vi "valves_pumpsteps.vi"(0 "COM4 in":refnum<k24>, 2 "Pump frequency":dbl=1.0, 3 "Commands in":T1, 5 "error in":errorcluster) -> (6 "COM4 out":refnum<k24>, 8 "error out":errorcluster)   [LabVIEW 2018]
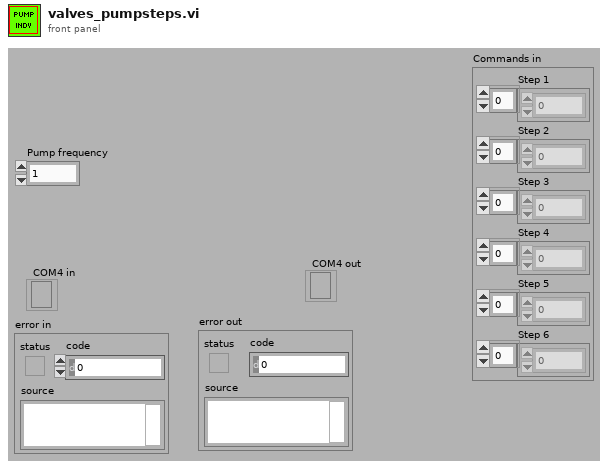
[diagram p1: front panel]
types:
  T1 = cluster{"Step 1":u8[], "Step 2":u8[], "Step 3":u8[], "Step 4":u8[], "Step 5":u8[], "Step 6":u8[]}
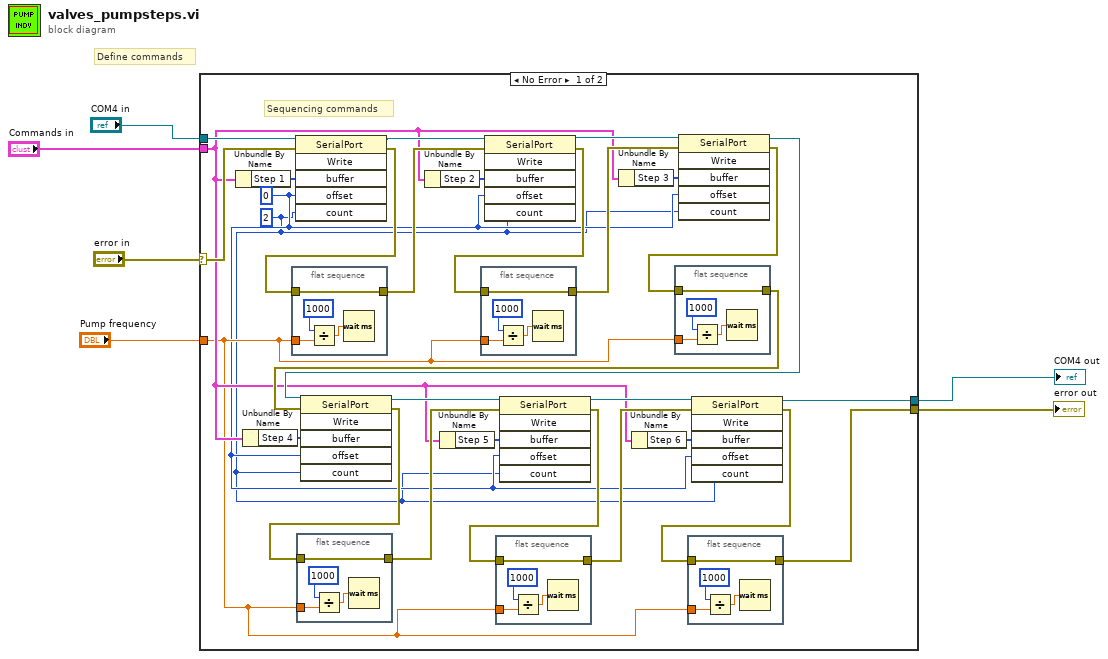
[diagram p0: block diagram]
diagram:
  # "Define commands"
  n1 = case shown="No Error" "error in" {
    selector: "error in" -> [w35 w62]
    tunnel: "COM4 in" -> [w36 w61]
    tunnel: [w15 w62] -> w2
    tunnel: "Commands in" -> [w17 _]
    tunnel: "Pump frequency" -> [w16 _]
    tunnel: [w23 w61] -> w3
    frame No Error {
      w7 = 2 ("count")
      w8 = 0 ("offset")
      # "Sequencing commands"
      n2 = Unbundle By Name(w17) -> ("Step 1"=w14:u8[])
      n3 = Unbundle By Name(w17) -> ("Step 4"=w11:u8[])
      n4 = flat-sequence {
        tunnel: [w60] -> w22
        tunnel: w34 -> [w60]
        tunnel: w16 -> [w58]
        frame #0 {
          n5 = Divide(x=u32 1000 ("milliseconds to wait"), y=w58) -> (x/y=w57:dbl)
          n6 = Wait (ms)(milliseconds to wait=w57) -> ()  [unwired: 1 out]
        }
      }
      n7 = invoke class="SerialPort" method="Write"(reference=w36, error in=w35, "buffer"=w14, "offset"=w8, "count"=w7) -> (reference out=w28:refnum<k24>, error out=w34:errorcluster)  [unwired: 1 in, 4 out]
      n8 = flat-sequence {
        tunnel: [w48] -> w19
        tunnel: w31 -> [w48]
        tunnel: w16 -> [w46]
        frame #0 {
          n9 = Divide(x=u32 1000 ("milliseconds to wait"), y=w46) -> (x/y=w45:dbl)
          n10 = Wait (ms)(milliseconds to wait=w45) -> ()  [unwired: 1 out]
        }
      }
      n11 = Unbundle By Name(w17) -> ("Step 2"=w13:u8[])
      n12 = Unbundle By Name(w17) -> ("Step 5"=w10:u8[])
      n13 = flat-sequence {
        tunnel: [w56] -> w21
        tunnel: w33 -> [w56]
        tunnel: w16 -> [w54]
        frame #0 {
          n14 = Divide(x=u32 1000 ("milliseconds to wait"), y=w54) -> (x/y=w53:dbl)
          n15 = Wait (ms)(milliseconds to wait=w53) -> ()  [unwired: 1 out]
        }
      }
      n16 = invoke class="SerialPort" method="Write"(reference=w28, error in=w22, "buffer"=w13, "offset"=w8, "count"=w7) -> (reference out=w27:refnum<k24>, error out=w33:errorcluster)  [unwired: 1 in, 4 out]
      n17 = flat-sequence {
        tunnel: [w44] -> w18
        tunnel: w30 -> [w44]
        tunnel: w16 -> [w42]
        frame #0 {
          n18 = Divide(x=u32 1000 ("milliseconds to wait"), y=w42) -> (x/y=w41:dbl)
          n19 = Wait (ms)(milliseconds to wait=w41) -> ()  [unwired: 1 out]
        }
      }
      n20 = Unbundle By Name(w17) -> ("Step 3"=w12:u8[])
      n21 = Unbundle By Name(w17) -> ("Step 6"=w9:u8[])
      n22 = flat-sequence {
        tunnel: [w52] -> w20
        tunnel: w32 -> [w52]
        tunnel: w16 -> [w50]
        frame #0 {
          n23 = Divide(x=u32 1000 ("milliseconds to wait"), y=w50) -> (x/y=w49:dbl)
          n24 = Wait (ms)(milliseconds to wait=w49) -> ()  [unwired: 1 out]
        }
      }
      n25 = invoke class="SerialPort" method="Write"(reference=w27, error in=w21, "buffer"=w12, "offset"=w8, "count"=w7) -> (reference out=w26:refnum<k24>, error out=w32:errorcluster)  [unwired: 1 in, 4 out]
      n26 = invoke class="SerialPort" method="Write"(reference=w26, error in=w20, "buffer"=w11, "offset"=w8, "count"=w7) -> (reference out=w25:refnum<k24>, error out=w31:errorcluster)  [unwired: 1 in, 4 out]
      n27 = invoke class="SerialPort" method="Write"(reference=w25, error in=w19, "buffer"=w10, "offset"=w8, "count"=w7) -> (reference out=w24:refnum<k24>, error out=w30:errorcluster)  [unwired: 1 in, 4 out]
      n28 = flat-sequence {
        tunnel: [w40] -> w15
        tunnel: w29 -> [w40]
        tunnel: w16 -> [w38]
        frame #0 {
          n29 = Divide(x=u32 1000 ("milliseconds to wait"), y=w38) -> (x/y=w37:dbl)
          n30 = Wait (ms)(milliseconds to wait=w37) -> ()  [unwired: 1 out]
        }
      }
      n31 = invoke class="SerialPort" method="Write"(reference=w24, error in=w18, "buffer"=w9, "offset"=w8, "count"=w7) -> (reference out=w23:refnum<k24>, error out=w29:errorcluster)  [unwired: 1 in, 4 out]
    }
    frame Error {
    }
  }
  "error out" <- w2
  "COM4 out" <- w3
